vi "Send_NamedNumSetStrings.vi"(6 "HighPriority (F)":bool, 8 "error in":errorcluster, 9 "NumericString":string[](array[string]), 10 "Control Label":string, 11 "Queue in":refnum<queue>) -> (0 "error out":errorcluster)   [LabVIEW 2018, in "UI_Library.lvlib"]
uses:
  UI_Library.lvlib
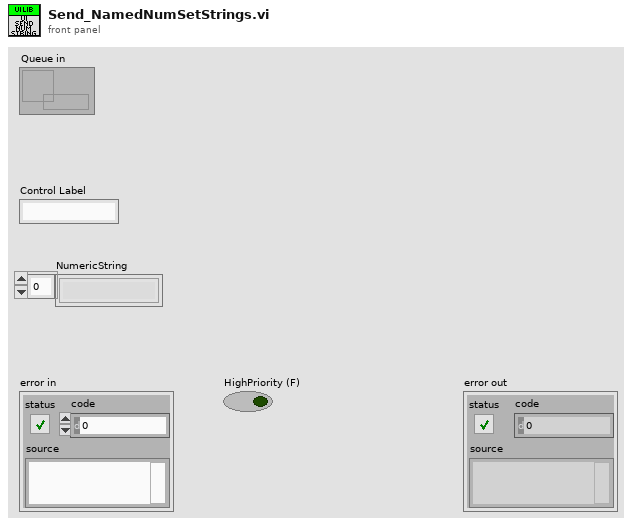
[diagram p1: front panel]
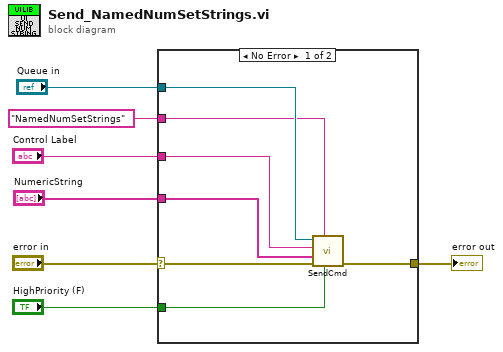
[diagram p0: block diagram]
diagram:
  n1 = case shown="No Error" "error in" {
    selector: "error in" -> [w13 w15]
    tunnel: "Queue in" -> [w14 _]
    tunnel: "Control Label" -> [w10 _]
    tunnel: "NumericString" -> [w9 _]
    tunnel: "NamedNumSetStrings" ("UICmd") -> [w11 _]
    tunnel: "HighPriority (F)" -> [w8 _]
    tunnel: [w12 w15] -> w7
    frame No Error {
      n2 = call "SendCmd.vi"("HighPriority (F)"=w8, "UICmd"=w11, "error in"=w13, "Control Data"=w9, "Control Label"=w10, "Queue in"=w14) -> ("error out"=w12:errorcluster)  [unwired: 5 in]
    }
    frame Error {
    }
  }
  "error out" <- w7
